vi "ambient_old.vi"() -> ()   [LabVIEW 2011]
panel:
  in  "MUTEX":bool
  out "standard output 2":string
  in  "Start Measurement":bool
  in  "QUIT":bool
  in  "KILL":bool
  in  "PAUSE":bool
  in  "RESUME":bool
  out "command":string
  out "standard error":string
  out "standard output":string
  # "Comandi di emergenza"
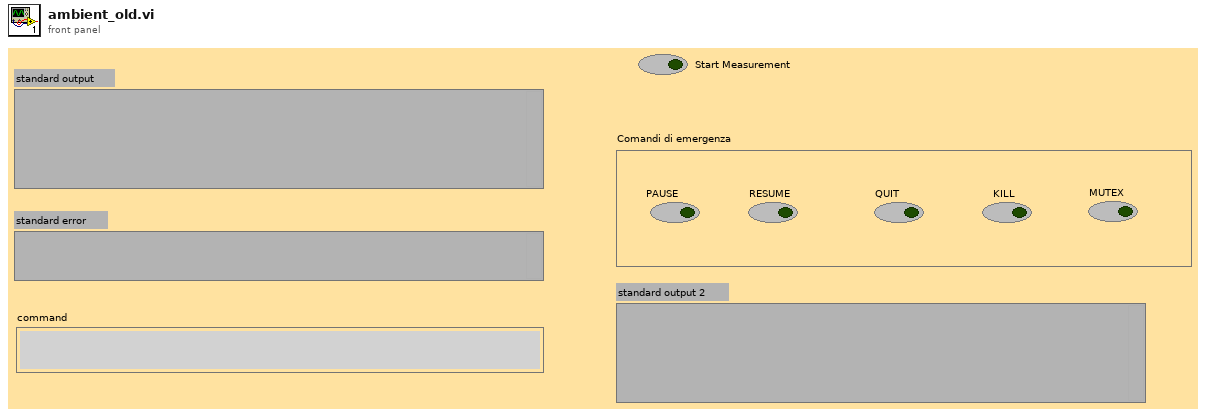
[diagram p1: front panel]
types:
  T1 = enum16{"open", "replace", "create", "open or create", "replace or create", "replace or create with confirmation"}
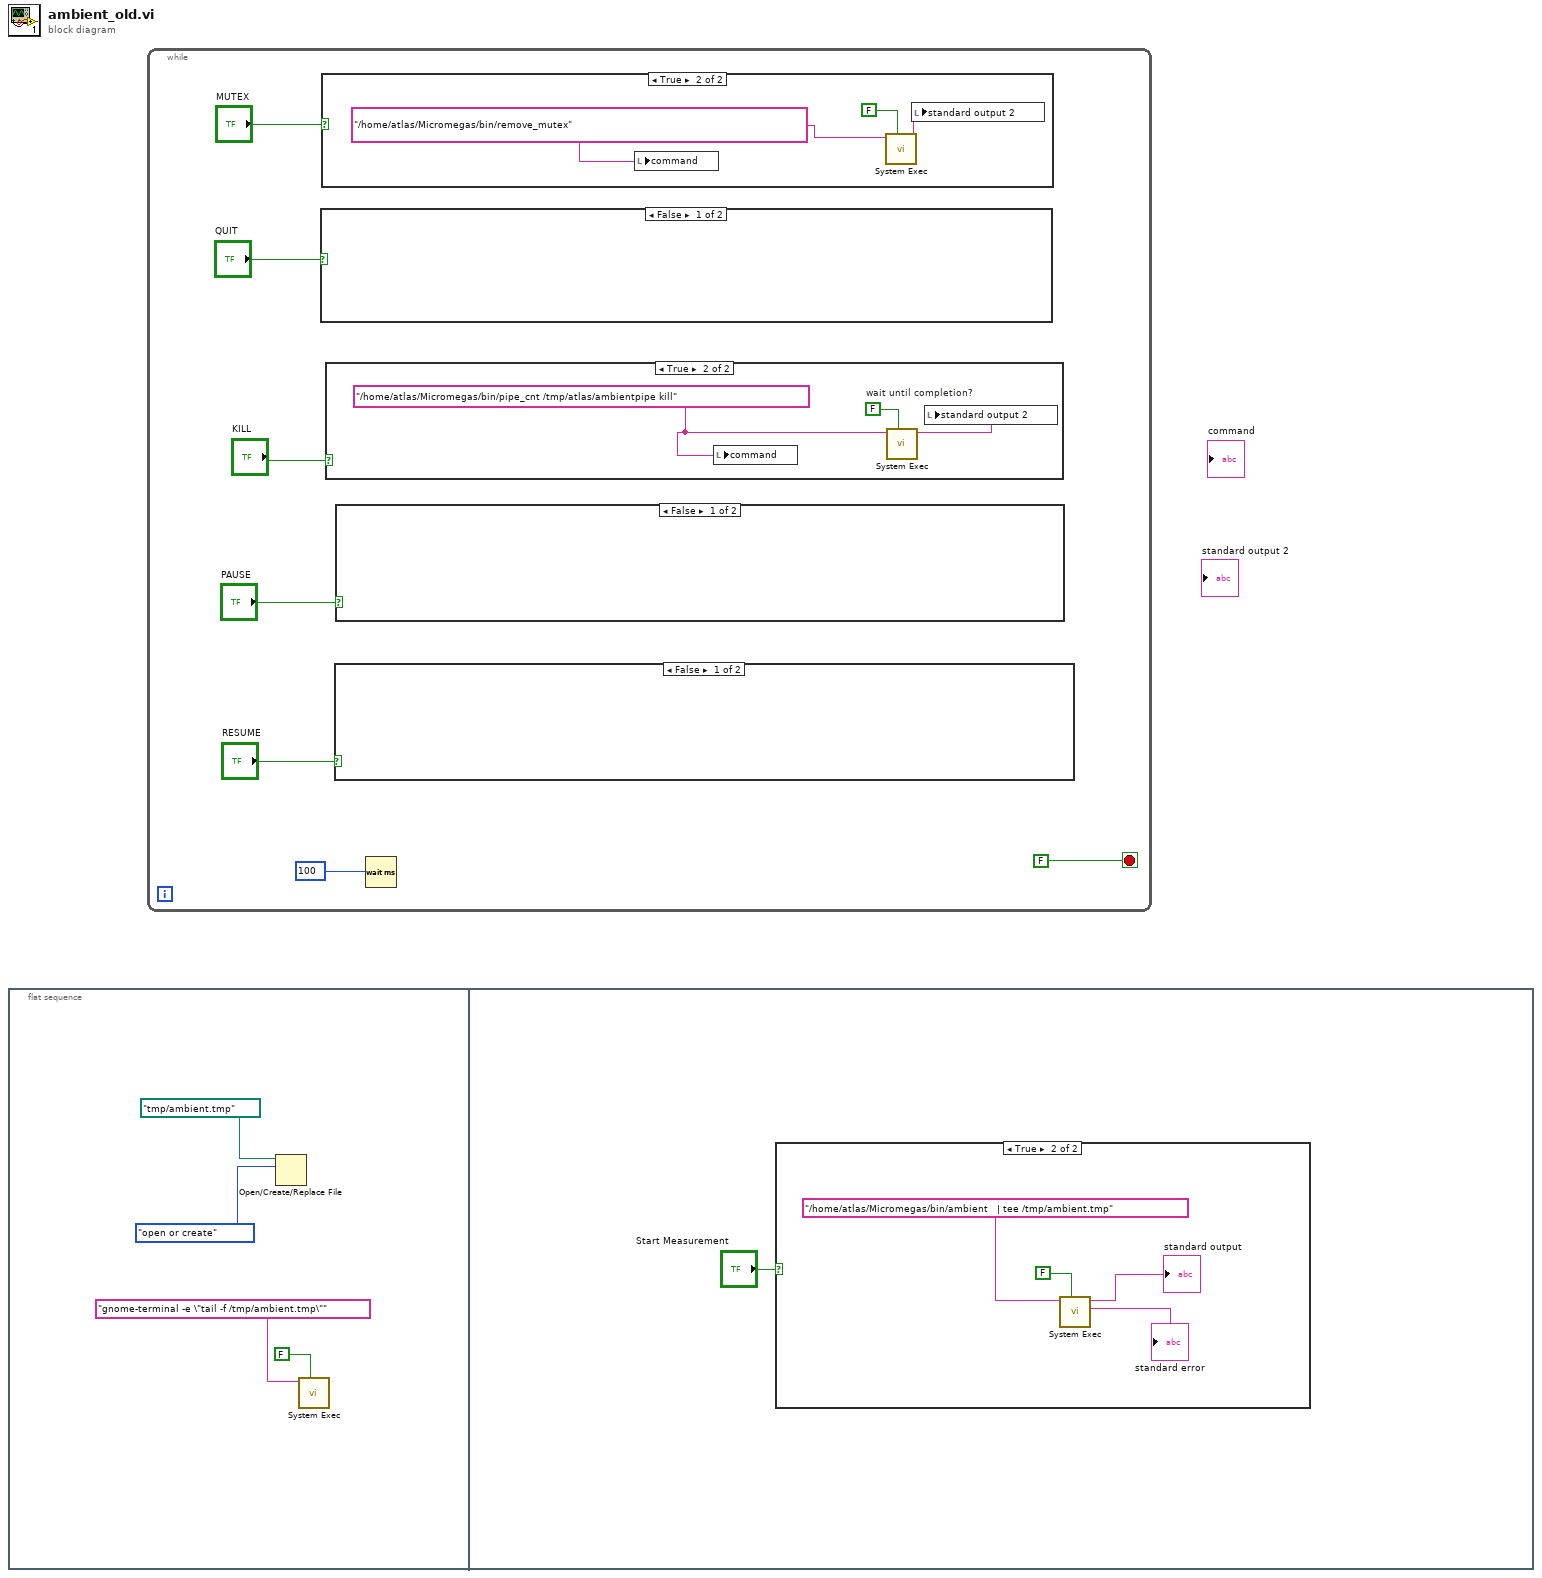
[diagram p0: block diagram]
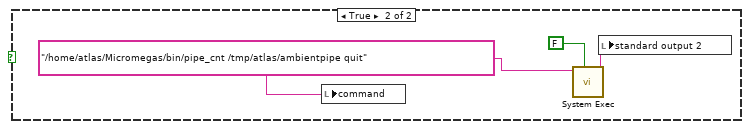
[diagram p4: hidden frame]
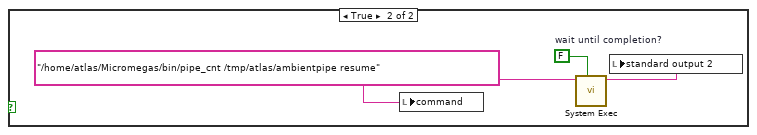
[diagram p5: hidden frame]
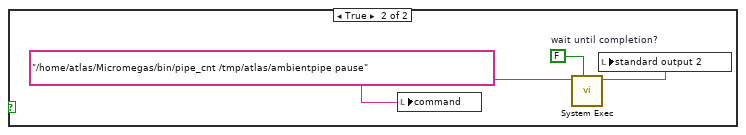
[diagram p6: hidden frame]
diagram:
  n1 = flat-sequence {
    frame #0 {
      n2 = Open/Create/Replace File(file path (use dialog)=path "/tmp/ambient.tmp", operation (0:open)=T1."open or create") -> ()  [unwired: 4 in, 3 out]
      n3 = call <vilib>:"System Exec.vi"("wait until completion? (T)"=FALSE, "command line"="gnome-terminal -e \"tail -f /tmp/ambient.tmp\"") -> ()  [unwired: 6 in, 4 out]
    }
    frame #1 {
      n4 = case shown="True" "Start Measurement" {
        frame False {
        }
        frame True {
          n5 = call <vilib>:"System Exec.vi"("wait until completion? (T)"=FALSE, "command line"="/home/atlas/Micromegas/bin/ambient   | tee /tmp/ambient.tmp") -> ("standard error"=→"standard error":string, "standard output"=→"standard output":string)  [unwired: 6 in, 2 out]
        }
      }
    }
  }
  n6 = while {
    stop <- FALSE ("stop") stop-if-true
    n7 = case shown="False" "QUIT" {
      frame False {
      }
      frame True {
        w21 = "/home/atlas/Micromegas/bin/pipe_cnt /tmp/atlas/ambientpipe quit" ("string")
        n8 = local write "command"(w21) -> ()
        n9 = call <vilib>:"System Exec.vi"("wait until completion? (T)"=FALSE, "command line"=w21) -> ("standard output"=w20:string)  [unwired: 6 in, 3 out]
        n10 = local write "standard output 2"(w20) -> ()
      }
    }
    n11 = case shown="True" "MUTEX" {
      frame False {
      }
      frame True {
        w18 = "/home/atlas/Micromegas/bin/remove_mutex" ("string")
        n12 = local write "command"(w18) -> ()
        n13 = call <vilib>:"System Exec.vi"("wait until completion? (T)"=FALSE, "command line"=w18) -> ("standard output"=w17:string)  [unwired: 6 in, 3 out]
        n14 = local write "standard output 2"(w17) -> ()
      }
    }
    n15 = case shown="True" "KILL" {
      frame False {
      }
      frame True {
        w29 = "/home/atlas/Micromegas/bin/pipe_cnt /tmp/atlas/ambientpipe kill" ("string")
        w31 = FALSE  # wait until completion?
        n16 = local write "command"(w29) -> ()
        n17 = call <vilib>:"System Exec.vi"("wait until completion? (T)"=w31, "command line"=w29) -> ("standard output"=w30:string)  [unwired: 6 in, 3 out]
        n18 = local write "standard output 2"(w30) -> ()
      }
    }
    n19 = case shown="False" "RESUME" {
      frame False {
      }
      frame True {
        w24 = "/home/atlas/Micromegas/bin/pipe_cnt /tmp/atlas/ambientpipe resume" ("string")
        w25 = FALSE  # wait until completion?
        n20 = local write "command"(w24) -> ()
        n21 = call <vilib>:"System Exec.vi"("wait until completion? (T)"=w25, "command line"=w24) -> ("standard output"=w23:string)  [unwired: 6 in, 3 out]
        n22 = local write "standard output 2"(w23) -> ()
      }
    }
    n23 = case shown="False" "PAUSE" {
      frame False {
      }
      frame True {
        w27 = "/home/atlas/Micromegas/bin/pipe_cnt /tmp/atlas/ambientpipe pause" ("string")
        w28 = FALSE  # wait until completion?
        n24 = local write "command"(w27) -> ()
        n25 = call <vilib>:"System Exec.vi"("wait until completion? (T)"=w28, "command line"=w27) -> ("standard output"=w26:string)  [unwired: 6 in, 3 out]
        n26 = local write "standard output 2"(w26) -> ()
      }
    }
    n27 = Wait (ms)(milliseconds to wait=100) -> ()  [unwired: 1 out]
  }
